vi "TEST File Loader.vi"() -> ()   [LabVIEW 2020]
uses:
  <userlib>/_NEVSTOP/Communicable State Machine(CSM)/addons/MassData-Parameter/Utility/Def-MassData Status Indicator(Vertical).ctl
  74f88484-48eb-4a50-b64a-67fdb578da88.vi
  88e3f29a-7662-4bb4-ab02-85fae349ecc4.vi
  <userlib>/_NEVSTOP/Communicable State Machine(CSM)/_Support/FGV-BroadcastRegistry/global-CSMQ FGV Change Flag.vi
  <userlib>/_NEVSTOP/Communicable State Machine(CSM)/_Support/CSMQ/_CSMOFGV.vi
  <userlib>/_NEVSTOP/Communicable State Machine(CSM)/addons/MassData-Parameter/CSM MassData Parameter Support.lvlib
  <userlib>/_NEVSTOP/Communicable State Machine(CSM)/Communicable State Machine.lvlib
  <userlib>/_NEVSTOP/Communicable State Machine(CSM)/addons/Watchdog/CSM Watchdog.lvlib
panel:
  in  "start":bool
  in  "stop":bool
  out "x-y":dbl
  in  "MassData Status":T1 {"r" scale=1.0..100000000.0 scale format="%#_6p"; "w" scale=1.0..100000000.0 scale format="%#_6p"}
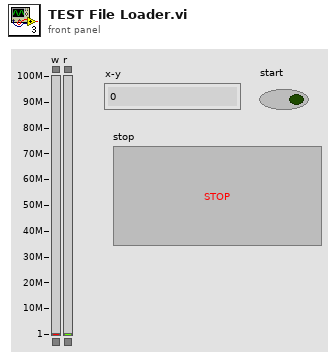
[diagram p1: front panel]
types:
  T1 = typedef "Def-MassData Status Indicator(Vertical).ctl" = cluster{"w":cluster{dbl, dbl}, "r":cluster{dbl, dbl}}
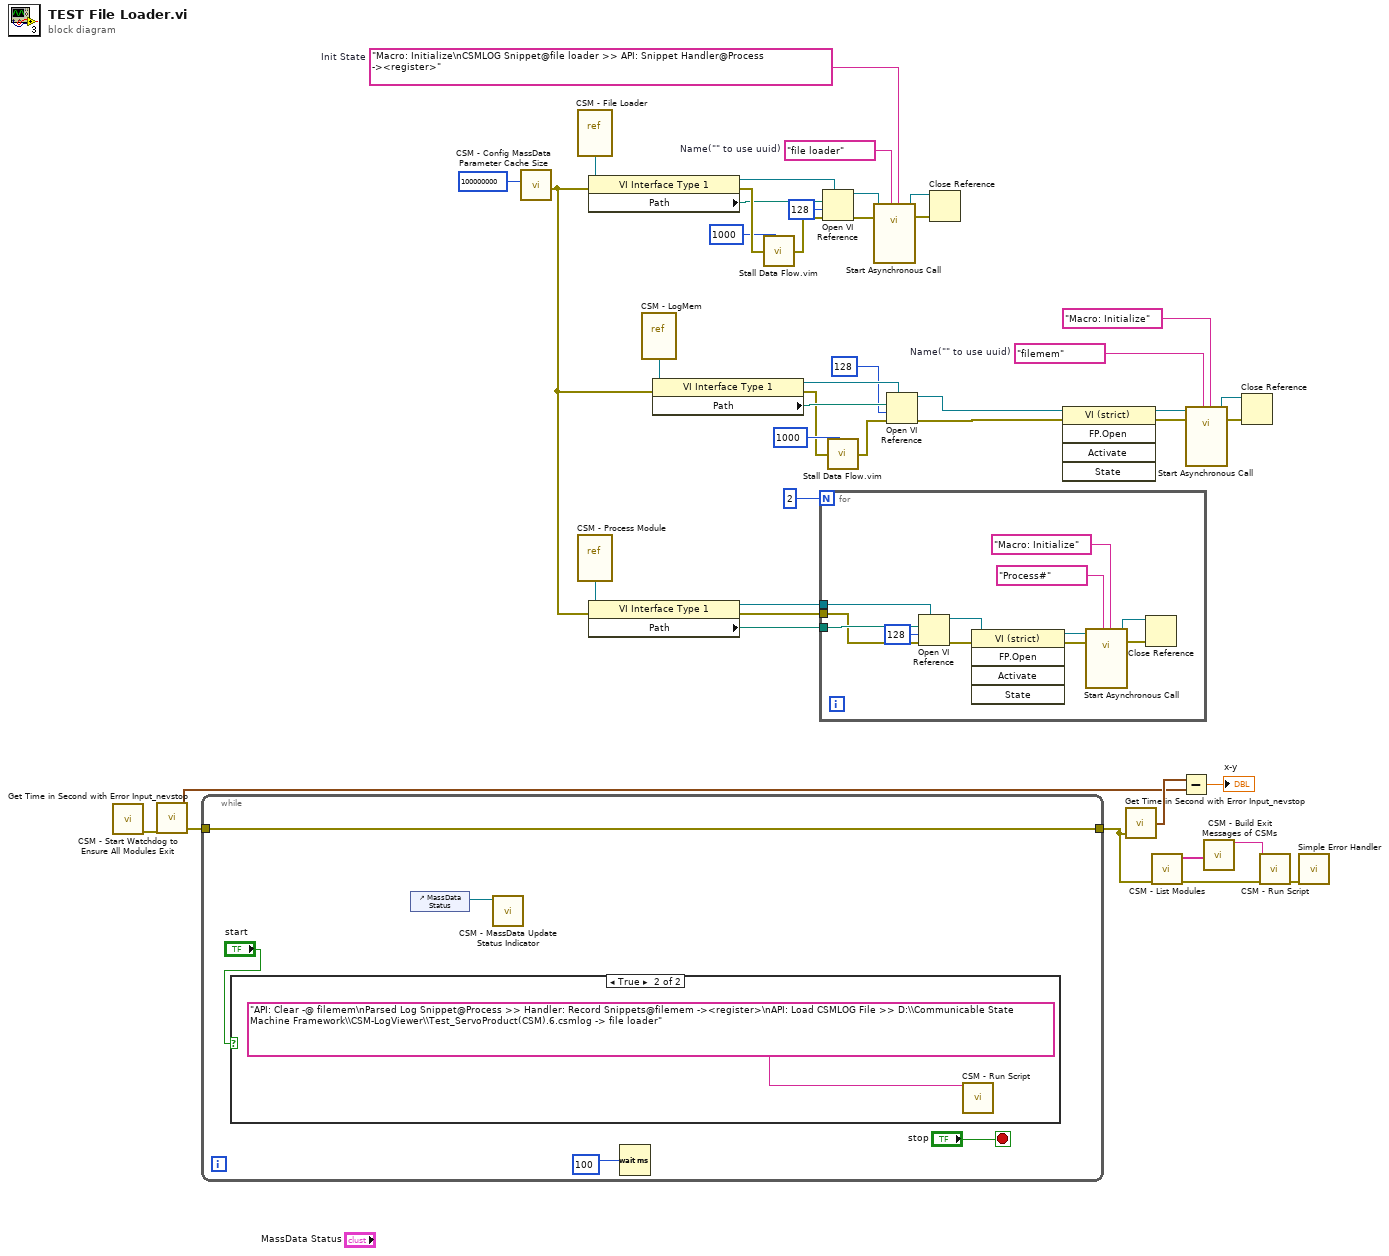
[diagram p0: block diagram]
diagram:
  w11 = "filemem"  # Name("" to use uuid)
  w35 = "Macro: Initialize\nCSMLOG Snippet@file loader >> API: Snippet Handler@Process -><register>"  # Init State
  w42 = "file loader"  # Name("" to use uuid)
  n1 = call <userlib>:"CSM - Start Watchdog to Ensure All Modules Exit.vi"() -> ("error out"=w1:errorcluster)  [unwired: 11 in]
  n2 = call <userlib>:"Get Time in Second with Error Input_nevstop.vi"("Error in"=w1) -> ("Error out"=w33:errorcluster, "current time"=w31:timestamp)  [unwired: 3 in]
  n3 = while {
    tunnel: [w48] -> w21
    tunnel: w33 -> [w48]
    stop <- "stop" stop-if-true
    n4 = case shown="True" "start" {
      frame False {
      }
      frame True {
        n5 = call <userlib>:"CSM - Run Script.vi"("single-line text"="API: Clear -@ filemem\nParsed Log Snippet@Process >> Handler: Record Snippets@filemem -><register>\nAPI: Load CSMLOG File >> D:\\Communicable State Machine Framework\\CSM-LogViewer\\Test_ServoProduct(CSM).6.csmlog -> file loader") -> ()  [unwired: 13 in, 2 out]
      }
    }
    n6 = control-ref of="MassData Status"() -> (w49:refnum<vi>)
    n7 = call <userlib>:"CSM - MassData Update Status Indicator.vi"("MassData Status Indicator"=w49) -> ()  [unwired: 10 in, 1 out]
    n8 = Wait (ms)(milliseconds to wait=u32 100) -> ()  [unwired: 1 out]
  }
  n9 = call <userlib>:"CSM - Config MassData Parameter Cache Size.vi"("size(1M)"=100000000) -> ("Error out"=w7:errorcluster)  [unwired: 10 in]
  n10 = vi-ref "CSM - File Loader.vi"() -> (w37:refnum<vi>)
  n11 = vi-ref "CSM - Process Module.vi"() -> (w29:refnum<vi>)
  n12 = property class="VI Interface Type 1"(reference=w37, error in=w7) -> (reference out=w41:refnum<vi>, error out=w39:errorcluster, "Path"=w38:path)
  n13 = property class="VI Interface Type 1"(reference=w29, error in=w7) -> (reference out=w26:refnum<vi>, error out=w27:errorcluster, "Path"=w28:path)
  n14 = vi-ref "CSM - LogMem.vi"() -> (w15:refnum<vi>)
  n15 = property class="VI Interface Type 1"(reference=w15, error in=w7) -> (reference out=w12:refnum<vi>, error out=w13:errorcluster, "Path"=w14:path)
  n16 = call "Stall Data Flow.vim"("value in"=w39, "milliseconds to wait"=u32 1000) -> ("value out"=w24:errorcluster)  [unwired: 1 out]
  n17 = for {
    N: 2 -> [_]
    tunnel: w28 -> [w62]
    tunnel: w27 -> [w61]
    tunnel: w26 -> [w60]
    n18 = Open VI Reference(type specifier VI Refnum (for type only)=w60, vi path=w62, options=128, error in (no error)=w61) -> (vi reference=w53:refnum<vi>, error out=w63:errorcluster)  [unwired: 2 in]
    n19 = invoke class="VI (strict)" method="FP.Open"(reference=w53, error in=w63) -> (reference out=w52:refnum<vi>, error out=w54:errorcluster)  [unwired: 3 in, 3 out]
    n20 = call-by-ref "Start Asynchronous Call"(reference=w52, error in=w54, "Init State(\"Macro: Initialize\")"="Macro: Initialize" ("Init State(\"Macro: Initialize\")"), "Name(\"\" to use uuid)"="Process#" ("Name(\"\" to use uuid)")) -> (reference out=w57:refnum<vi>, error out=w58:errorcluster)  [unwired: 10 in]
    n21 = Close Reference(reference=w57, error in (no error)=w58) -> ()  [unwired: 1 out]
  }
  n22 = Open VI Reference(type specifier VI Refnum (for type only)=w41, vi path=w38, options=128, error in (no error)=w24) -> (vi reference=w40:refnum<vi>, error out=w36:errorcluster)  [unwired: 2 in]
  n23 = call "Stall Data Flow.vim"("value in"=w13, "milliseconds to wait"=u32 1000) -> ("value out"=w16:errorcluster)  [unwired: 1 out]
  n24 = call-by-ref "Start Asynchronous Call"(reference=w40, error in=w36, "Init State(\"Macro: Initialize\")"=w35, "Name(\"\" to use uuid)"=w42) -> (reference out=w44:refnum<vi>, error out=w43:errorcluster)  [unwired: 10 in]
  n25 = Open VI Reference(type specifier VI Refnum (for type only)=w12, vi path=w14, options=128, error in (no error)=w16) -> (vi reference=w5:refnum<vi>, error out=w6:errorcluster)  [unwired: 2 in]
  n26 = Close Reference(reference=w44, error in (no error)=w43) -> ()  [unwired: 1 out]
  n27 = invoke class="VI (strict)" method="FP.Open"(reference=w5, error in=w6) -> (reference out=w4:refnum<vi>, error out=w3:errorcluster)  [unwired: 3 in, 3 out]
  n28 = call <userlib>:"Get Time in Second with Error Input_nevstop.vi"("Error in"=w21) -> ("current time"=w32:timestamp)  [unwired: 3 in, 1 out]
  n29 = call <userlib>:"CSM - List Modules.vi"("Error in"=w21) -> ("Error out"=w19:errorcluster, "Module Names"=w22:string[])  [unwired: 9 in]
  n30 = Subtract(x=w32, y=w31) -> (x-y=→"x-y":dbl)
  n31 = call-by-ref "Start Asynchronous Call"(reference=w4, error in=w3, "Init State(\"Macro: Initialize\")"="Macro: Initialize" ("Init State(\"Macro: Initialize\")"), "Name(\"\" to use uuid)"=w11) -> (reference out=w9:refnum<vi>, error out=w10:errorcluster)  [unwired: 10 in]
  n32 = call <userlib>:"CSM - Build Exit Messages of CSMs.vi"("CSMs"=w22) -> ("States"=w20:string)  [unwired: 14 in]
  n33 = Close Reference(reference=w9, error in (no error)=w10) -> ()  [unwired: 1 out]
  n34 = call <userlib>:"CSM - Run Script.vi"("single-line text"=w20, "error in (no error)"=w19) -> ("error out"=w18:errorcluster)  [unwired: 12 in, 1 out]
  n35 = call <vilib>:"Simple Error Handler.vi"("error in (no error)"=w18) -> ()  [unwired: 4 in, 5 out]
